vi "Get Fourier Series of Signal.vi"(10 "N":dbl, 11 "Signal":cdb[](array[numeric])) -> (3 "Coefficients":cdb[](array[numeric]))   [LabVIEW 2020]
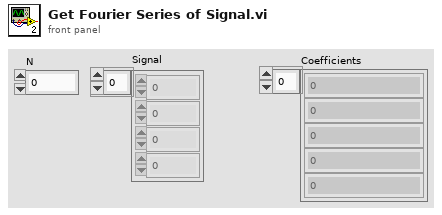
[diagram p1: front panel]
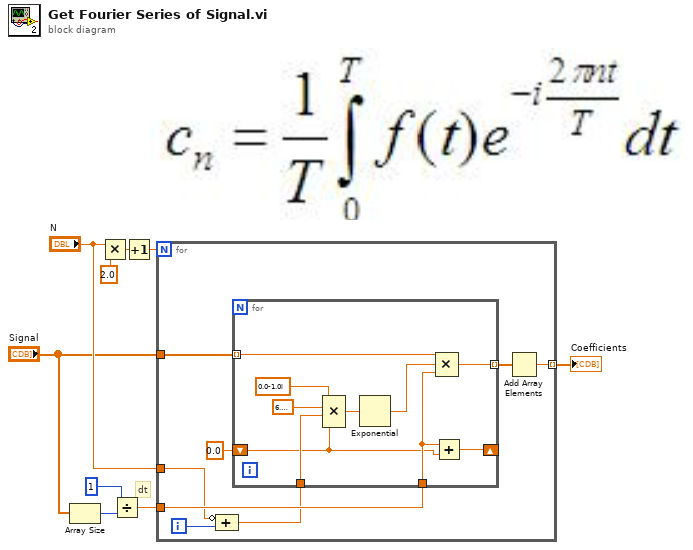
[diagram p0: block diagram]
diagram:
  # "dt"
  n1 = Array Size(array="Signal") -> (size(s)=w9:i32)
  n2 = Multiply(x="N", y=2.0) -> (x*y=w5:dbl)
  n3 = Divide(x=1, y=w9) -> (x/y=w8:dbl)
  n4 = Increment(x=w5) -> (x+1=w4:dbl)
  n5 = for {
    N: w4 -> [_]
    tunnel: "Signal" -> [w17]
    tunnel: w8 -> [w16]
    tunnel: [w10] -> w7 mode=indexing
    tunnel: "N" -> [w14]
    i -> [w13]
    n6 = Compound Arithmetic op=unknown(invert w14, w13) -> (w12:dbl)
    n7 = for {
      tunnel: w17 -> [w25] mode=indexing
      tunnel: w12 -> [w26]
      tunnel: w16 -> [w21]
      tunnel: [w23] -> w15 mode=indexing
      shift-right: [w22] -> _
      shift-left: 0.0 -> [w20]
      n8 = Compound Arithmetic op=MULTIPLY(cdb 0.0-1.0i, 6.283185307179586, w26, w20) -> (w27:cdb)
      n9 = Exponential(1:w27) -> (0:w24:cdb)
      n10 = Add(x=w21, y=w20) -> (x+y=w22:dbl)
      n11 = Compound Arithmetic op=MULTIPLY(w25, w24, w21) -> (w23:cdb)
    }
    n12 = Add Array Elements(numeric array=w15) -> (sum=w10:cdb)
  }
  "Coefficients" <- w7
